vi "SetMode.vi"(8 "error in (no error)":errorcluster, 9 "custom blink":T2, 10 "mode":T1, 11 "Qbus in":refnum<class "Qbus.lvclass">) -> (0 "error out":errorcluster, 3 "Qbus out":refnum<class "Qbus.lvclass">)   [LabVIEW 2017, in "BlinkProcess.lvlib"]
doc: "Sets the blinking pattern of the USER1 LED."
uses:
  <vilib>/addons/BlinkProcess/BlinkProcess.lvlib
  <vilib>/addons/BlinkProcess/controls/customBlinkConfig.ctl
  <vilib>/addons/BlinkProcess/controls/mode.ctl
  <vilib>/addons/Qbus/Qbus.lvclass
  <vilib>/addons/BlinkProcess/controls/ModeConfig.ctl
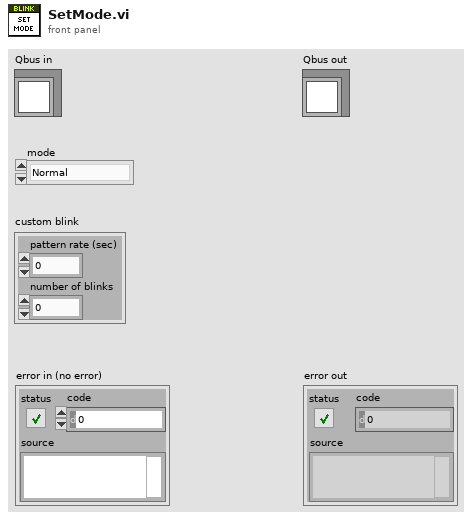
[diagram p1: front panel]
types:
  T1 = typedef "BlinkProcess.lvlib/mode.ctl" = enum16{"Normal", "Error", "On", "Off", "Custom"}
  T2 = typedef "BlinkProcess.lvlib/customBlinkConfig.ctl" = cluster{"pattern rate (sec)":dbl, "number of blinks":u32}
  T3 = typedef "BlinkProcess.lvlib/ModeConfig.ctl" = cluster{"mode":T1, "custom blink":T2}
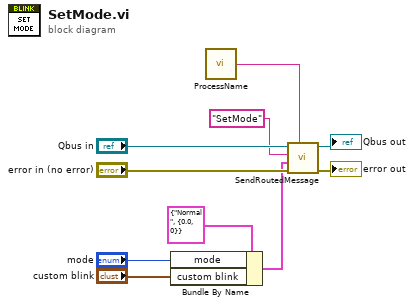
[diagram p0: block diagram]
diagram:
  n1 = Bundle By Name(cluster=T3 {"mode"=enum."Normal", "custom blink"={"pattern rate (sec)"=0.0, "number of blinks"=0}} ("Mode Config"), "mode"="mode", "custom blink"="custom blink") -> (w4:T3)
  n2 = call <vilib>:"ProcessName.vi"() -> ("process name"=w6:string)  [unwired: 5 in]
  n3 = call <vilib>:"SendRoutedMessage.vi"("listener process"=w6, "error in (no error)"="error in (no error)", "message value"=w4, "message name"="SetMode" ("MsgName"), "Qbus in"="Qbus in") -> ("error in (no error)"=→"error out":errorcluster, "Qbus out"=→"Qbus out":refnum<class "Qbus.lvclass">)  [unwired: 5 in]
